vi "Read Column index.vi"(11 "Series in":refnum<class "Series.lvclass">) -> (2 "Column index":i32=-1, 3 "Series out":refnum<class "Series.lvclass">)   [LabVIEW 2017]
uses:
  Series.lvclass
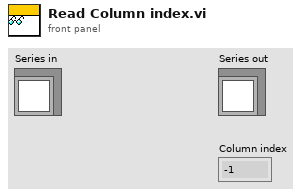
[diagram p1: front panel]
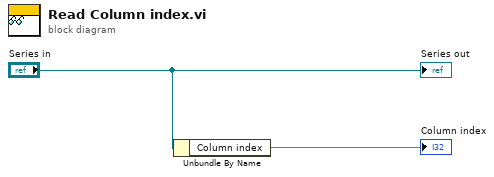
[diagram p0: block diagram]
diagram:
  n1 = Unbundle By Name("Series in") -> ("Column index"=→"Column index")
  "Series out" <- "Series in"
